vi "WebSocket Read.vi"(8 "error in (no error)":errorcluster, 9 "timeout ms (5000)":i32=5000, 11 "WebSocket Connection in":refnum<k5>) -> (0 "error out":errorcluster, 1 "Opcode":u8, 2 "Data":string, 3 "WebSocket Connection out":refnum<k5>)   [LabVIEW 2018]
doc: "Reads and decodes an incoming WebSockets message.\nWebSockets API 1.3.0.13\nSam Sharp - Intelligent Energy\nCopyright (c) 2015, Intelligent Energy"
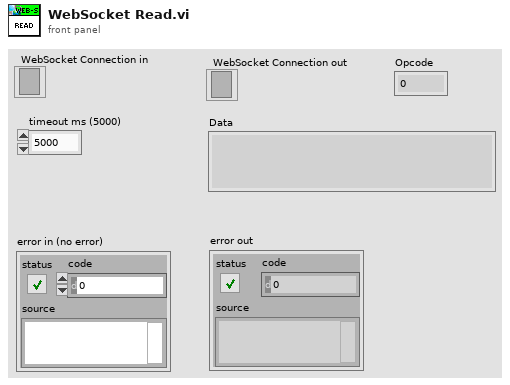
[diagram p1: front panel]
types:
  T1 = enum16{"big-endian, network order", "native, host order", "little-endian"}
  T2 = enum16{"Standard", "Buffered", "CRLF", "Immediate"}
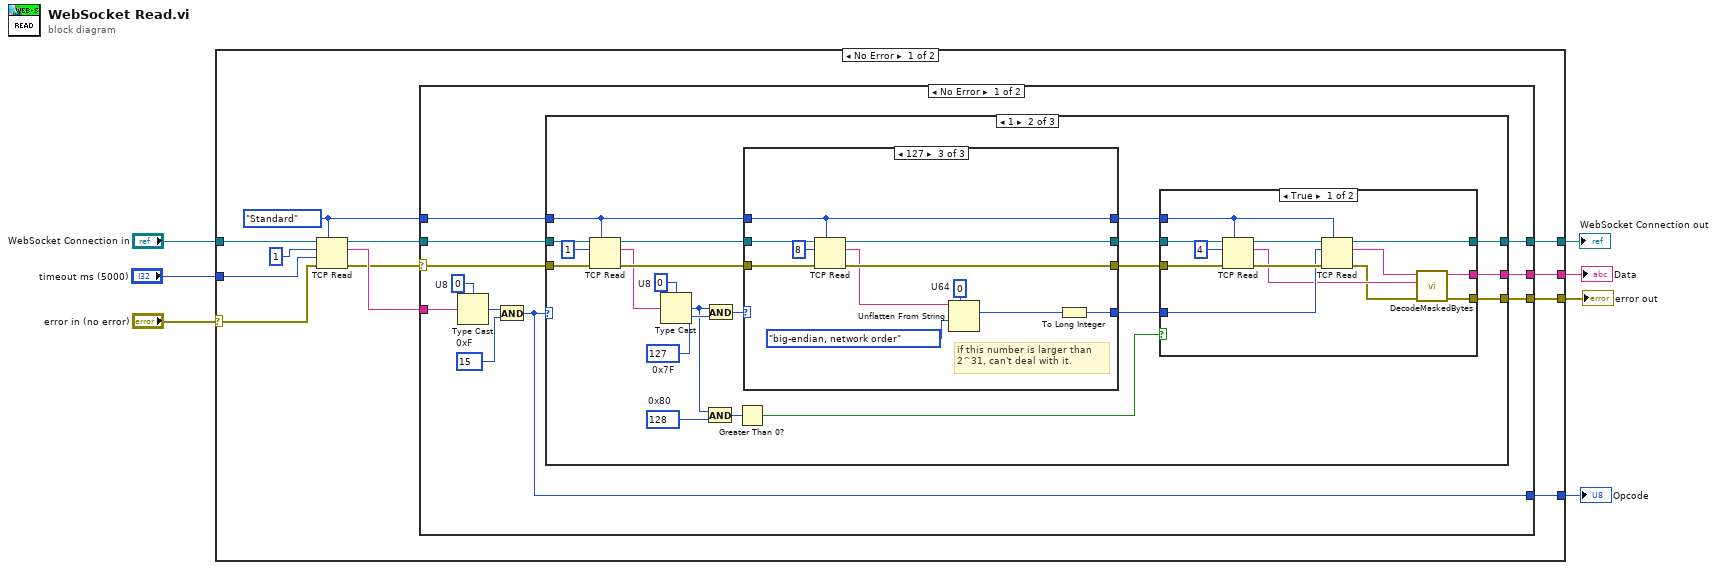
[diagram p0: block diagram]
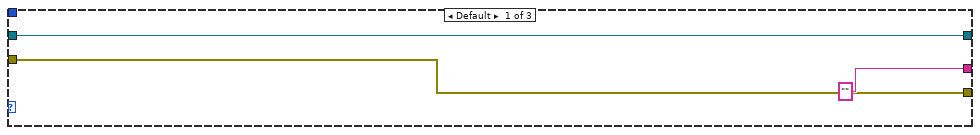
[diagram p2: hidden frame]
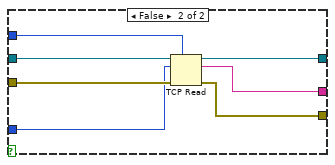
[diagram p3: hidden frame]
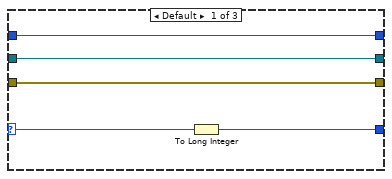
[diagram p4: hidden frame]
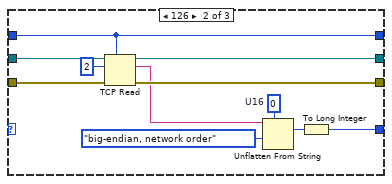
[diagram p5: hidden frame]
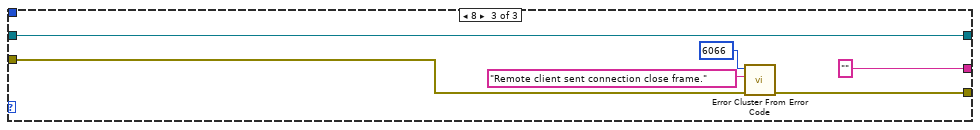
[diagram p6: hidden frame]
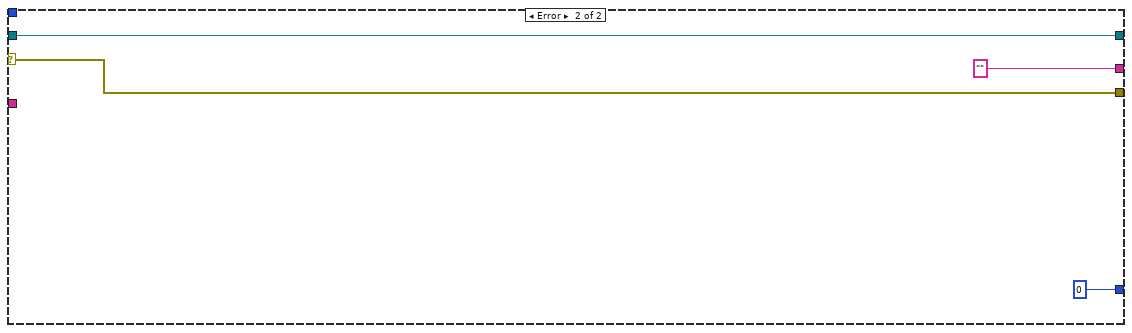
[diagram p7: hidden frame]
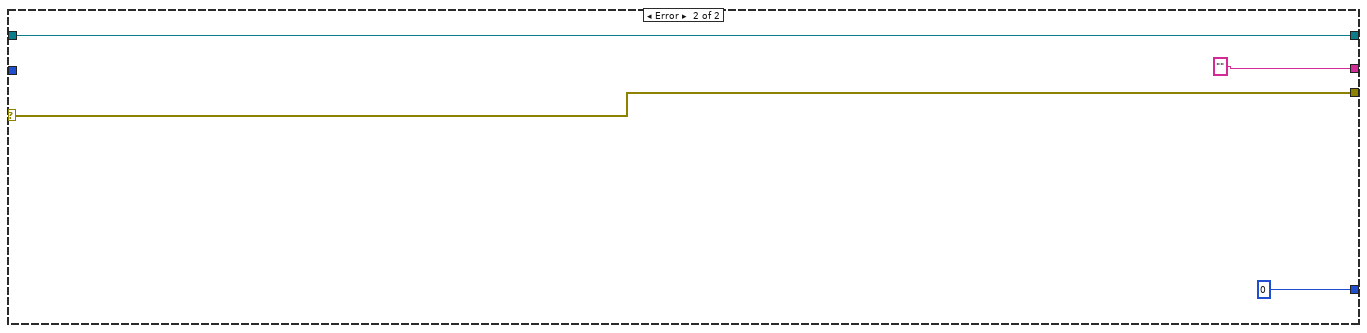
[diagram p8: hidden frame]
diagram:
  n1 = case shown="No Error" "error in (no error)" {
    selector: "error in (no error)" -> [w13 w115]
    tunnel: "WebSocket Connection in" -> [w19 w114]
    tunnel: [w14 w114] -> w6
    tunnel: [w12 "" ("data out")] -> w5
    tunnel: [w11 w115] -> w3
    tunnel: "timeout ms (5000)" -> [w10 _]
    tunnel: [w8 u8 0] -> w1
    frame No Error {
      w15 = T2."Standard" ("mode (standard)")
      n2 = TCP Read(connection ID=w19, bytes to read=1, error in (no error)=w13, 7:w15, 9:w10) -> (connection ID out=w16:refnum<k5>, data out=w17:string, error out=w9:errorcluster)
      n3 = case shown="No Error" w9 {
        selector: w9 -> [w25 w109]
        tunnel: w17 -> [w24 _]
        tunnel: w16 -> [w30 w111]
        tunnel: w15 -> [w29 _]
        tunnel: [w28 w111] -> w14
        tunnel: [w27 "" ("Decoded Data")] -> w12
        tunnel: [w26 w109] -> w11
        tunnel: [w20 u8 0] -> w8
        frame No Error {
          w21 = u8 15  # 0xF
          w23 = u8 0  # U8
          n4 = Type Cast(type=w23, x=w24) -> (*(type *) &x=w22:u8)
          n5 = And(x=w22, y=w21) -> (x .and. y?=w20:u8)
          n6 = case shown="1" w20 {
            tunnel: w30 -> [w33 w45 w107]
            tunnel: w29 -> [_ w43 _]
            tunnel: [w33 w54 w107] -> w28
            tunnel: ["" ("Decoded Data") w47 "" ("Decoded Data")] -> w27
            tunnel: [w31 w46 w105] -> w26
            tunnel: w25 -> [w31 w41 w104]
            frame Default {
            }
            frame 1 {
              w37 = u8 128  # 0x80
              w38 = u8 0  # U8
              w53 = u8 127  # 0x7F
              n7 = TCP Read(connection ID=w45, bytes to read=1, error in (no error)=w41, 7:w43) -> (connection ID out=w44:refnum<k5>, data out=w39:string, error out=w40:errorcluster)  [unwired: 1 in]
              n8 = Type Cast(type=w38, x=w39) -> (*(type *) &x=w36:u8)
              n9 = And(x=w36, y=w37) -> (x .and. y?=w35:u8)
              n10 = And(x=w36, y=w53) -> (x .and. y?=w52:u8)
              n11 = Greater Than 0?(x=w35) -> (x > 0?=w34:bool)
              n12 = case shown="127" w52 {
                selector: w52 -> [w78 _ _]
                tunnel: w44 -> [w79 w90 w100]
                tunnel: [w79 w89 w99] -> w51
                tunnel: w43 -> [w76 w87 w95]
                tunnel: [w77 w80 w98] -> w48
                tunnel: [w76 w87 w95] -> w50
                tunnel: [w75 w86 w97] -> w49
                tunnel: w40 -> [w75 w85 w96]
                frame Default {
                  n13 = To Long Integer(number=w78) -> (32bit integer=w77:i32)
                }
                frame 126 {
                  w84 = u16 0  # U16
                  n14 = TCP Read(connection ID=w90, bytes to read=2, error in (no error)=w85, 7:w87) -> (connection ID out=w89:refnum<k5>, data out=w82:string, error out=w86:errorcluster)  [unwired: 1 in]
                  n15 = Unflatten From String(type=w84, binary string=w82, byte order (0:big-endian, network order)=T1."big-endian, network order") -> (value=w81:u16)  [unwired: 2 in, 2 out]
                  n16 = To Long Integer(number=w81) -> (32bit integer=w80:i32)
                }
                frame 127 {
                  w94 = u64 0  # U64
                  # "if this number is larger than\n2^31, can't deal with it."
                  n17 = TCP Read(connection ID=w100, bytes to read=8, error in (no error)=w96, 7:w95) -> (connection ID out=w99:refnum<k5>, data out=w93:string, error out=w97:errorcluster)  [unwired: 1 in]
                  n18 = Unflatten From String(type=w94, binary string=w93, byte order (0:big-endian, network order)=T1."big-endian, network order") -> (value=w92:u64)  [unwired: 2 in, 2 out]
                  n19 = To Long Integer(number=w92) -> (32bit integer=w98:i32)
                }
              }
              n20 = case shown="True" w34 {
                tunnel: [w67 w74] -> w54
                tunnel: w51 -> [w66 w73]
                tunnel: w50 -> [w64 w72]
                tunnel: w49 -> [w63 w71]
                tunnel: w48 -> [w60 w70]
                tunnel: [w57 w68] -> w47
                tunnel: [w55 w69] -> w46
                frame True {
                  n21 = TCP Read(connection ID=w66, bytes to read=4, error in (no error)=w63, 7:w64) -> (connection ID out=w65:refnum<k5>, data out=w59:string, error out=w62:errorcluster)  [unwired: 1 in]
                  n22 = TCP Read(connection ID=w65, bytes to read=w60, error in (no error)=w62, 7:w64) -> (connection ID out=w67:refnum<k5>, data out=w58:string, error out=w56:errorcluster)  [unwired: 1 in]
                  n23 = call "DecodeMaskedBytes.vi"("error in (no error)"=w56, "Mask Bytes"=w59, "Encoded Data"=w58) -> ("error out"=w55:errorcluster, "Decoded Data"=w57:string)  [unwired: 7 in]
                }
                frame False {
                  n24 = TCP Read(connection ID=w73, bytes to read=w70, error in (no error)=w71, 7:w72) -> (connection ID out=w74:refnum<k5>, data out=w68:string, error out=w69:errorcluster)  [unwired: 1 in]
                }
              }
            }
            frame 8 {
              n25 = call <vilib>:"Error Cluster From Error Code.vi"("error in (no error)"=w104, "error message (\"\")"="Remote client sent connection close frame." ("error message (\"\")"), "error code (0)"=6066) -> ("error out"=w105:errorcluster)  [unwired: 6 in]
            }
          }
        }
        frame Error {
        }
      }
    }
    frame Error {
    }
  }
  "WebSocket Connection out" <- w6
  "Data" <- w5
  "error out" <- w3
  "Opcode" <- w1
